vi "Get Steering Frame Type from String.vi"(10 "dvr (F)":bool, 11 "steering type":string) -> (3 "data type":variant)   [LabVIEW 2017, in "NI_Robotics_Steering Class Types.lvlib"]
uses:
  <vilib>/robotics/Steering/Class Type Definitions/NI_Robotics_Steering Class Types.lvlib
  <vilib>/robotics/Steering/Class Type Definitions/Steering Frame.ctl
  <vilib>/robotics/Steering/Steering Frame/NI_Robotics_Steering Frame.lvclass
  <vilib>/robotics/Steering/Class Type Definitions/Steering Frame DVR.ctl
  <vilib>/robotics/Steering/Class Type Definitions/Differential Steering Frame.ctl
  <vilib>/robotics/Steering/Differential Steering Frame/NI_Robotics_Differential Steering Frame.lvclass
  <vilib>/robotics/Steering/Class Type Definitions/Differential Steering Frame DVR.ctl
  <vilib>/robotics/Steering/Class Type Definitions/Mecanum Steering Frame.ctl
  <vilib>/robotics/Steering/Mecanum Steering Frame/NI_Robotics_Mecanum Steering Frame.lvclass
  <vilib>/robotics/Steering/Class Type Definitions/Mecanum Steering Frame DVR.ctl
  <vilib>/robotics/Steering/Class Type Definitions/Ackermann Steering Frame.ctl
  <vilib>/robotics/Steering/Ackermann Steering Frame/NI_Robotics_Ackermann Steering Frame.lvclass
  <vilib>/robotics/Steering/Class Type Definitions/Ackermann Steering Frame DVR.ctl
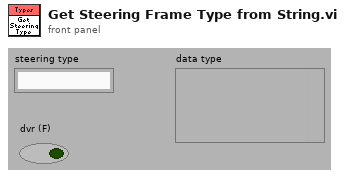
[diagram p1: front panel]
types:
  T1 = typedef "NI_Robotics_Steering Class Types.lvlib/Steering Frame.ctl" = refnum<class "NI_Robotics_Steering Frame.lvclass">
  T2 = typedef "NI_Robotics_Steering Class Types.lvlib/Steering Frame DVR.ctl" = refnum<data-value>
  T3 = typedef "NI_Robotics_Steering Class Types.lvlib/Differential Steering Frame.ctl" = refnum<class "NI_Robotics_Differential Steering Frame.lvclass">
  T4 = typedef "NI_Robotics_Steering Class Types.lvlib/Differential Steering Frame DVR.ctl" = refnum<data-value>
  T5 = typedef "NI_Robotics_Steering Class Types.lvlib/Mecanum Steering Frame.ctl" = refnum<class "NI_Robotics_Mecanum Steering Frame.lvclass">
  T6 = typedef "NI_Robotics_Steering Class Types.lvlib/Mecanum Steering Frame DVR.ctl" = refnum<data-value>
  T7 = typedef "NI_Robotics_Steering Class Types.lvlib/Ackermann Steering Frame.ctl" = refnum<class "NI_Robotics_Ackermann Steering Frame.lvclass">
  T8 = typedef "NI_Robotics_Steering Class Types.lvlib/Ackermann Steering Frame DVR.ctl" = refnum<data-value>
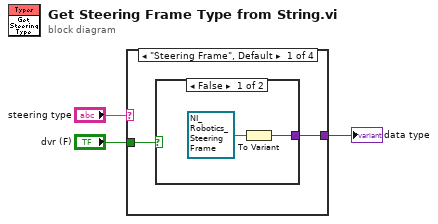
[diagram p0: block diagram]
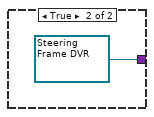
[diagram p2: hidden frame]
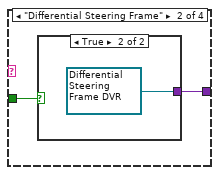
[diagram p3: hidden frame]
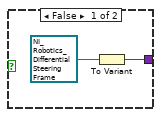
[diagram p4: hidden frame]
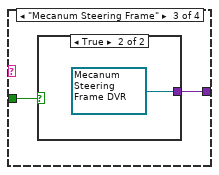
[diagram p5: hidden frame]
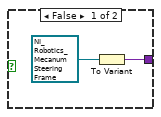
[diagram p6: hidden frame]
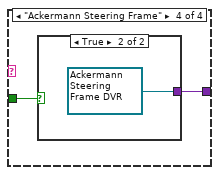
[diagram p7: hidden frame]
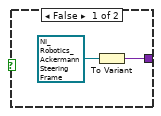
[diagram p8: hidden frame]
diagram:
  n1 = case shown="\"Steering Frame\", Default" "steering type" {
    tunnel: "dvr (F)" -> [w5 w10 w15 w20]
    tunnel: [w4 w9 w14 w19] -> w1
    frame "Steering Frame", Default {
      n2 = case shown="False" w5 {
        tunnel: [w6 T2 refnum ("steering frame ref")] -> w4
        frame False {
          n3 = To Variant(anything=T1 refnum ("steering frame")) -> (Variant=w6:variant)
        }
        frame True {
        }
      }
    }
    frame "Differential Steering Frame" {
      n4 = case shown="True" w10 {
        tunnel: [w12 T4 refnum ("differential steering frame ref")] -> w9
        frame False {
          n5 = To Variant(anything=T3 refnum ("differential steering frame")) -> (Variant=w12:variant)
        }
        frame True {
        }
      }
    }
    frame "Mecanum Steering Frame" {
      n6 = case shown="True" w15 {
        tunnel: [w17 T6 refnum ("mecanum steering frame ref")] -> w14
        frame False {
          n7 = To Variant(anything=T5 refnum ("mecanum steering frame")) -> (Variant=w17:variant)
        }
        frame True {
        }
      }
    }
    frame "Ackermann Steering Frame" {
      n8 = case shown="True" w20 {
        tunnel: [w22 T8 refnum ("ackermann steering frame ref")] -> w19
        frame False {
          n9 = To Variant(anything=T7 refnum ("ackermann steering frame")) -> (Variant=w22:variant)
        }
        frame True {
        }
      }
    }
  }
  "data type" <- w1
